vi "get Baud Rate.vi"(11 "port_num":i32) -> (3 "function return":i32)   [LabVIEW 2021, in "dxl_x86_c.lvlib"]
doc: "WINDECLSPEC int getBaudRate (int port_num);"
uses:
  dxl_x86_c.lvlib
  dxl_x86_c.dll
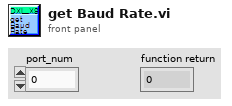
[diagram p1: front panel]
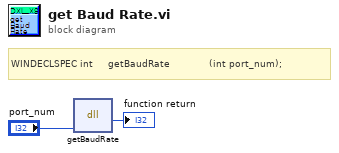
[diagram p0: block diagram]
diagram:
  # "WINDECLSPEC int     getBaudRate             (int port_num);"
  n1 = dll-call lib="C:/Users/ashek/Desktop/ashekim/ws/DynamixelSDK/labview/labview/dxl_x86_c.*" fn="getBaudRate"("port_num"="port_num") -> (→"function return":i32)  [unwired: 4 in, 2 out]
